vi "DestroyClone.vi"(8 "error in (no error)":errorcluster, 9 "Exit via Stop Module Req?":bool, 10 "Wait for Module to stop?":bool, 11 "ModuleAdmin":refnum<class "ModuleAdmin.lvclass">) -> (0 "error out":errorcluster, 1 "External Launch":bool, 3 "Mod Admin out":refnum<class "ModuleAdmin.lvclass">)   [LabVIEW 2014, in "SamplerModule.lvlib"]
uses:
  SamplerModule.lvlib
  <userlib>/NIST/ModuleAdminLib/ModuleAdmin/ModuleAdmin.lvclass
  <userlib>/NIST/ModuleAdminLib/ModuleAdmin/ModuleAdmin.lvclass/ModuleAdmin.ctl
  <userlib>/NIST/ModuleAdminLib/ModuleAdmin/Accessors/Read CloneRegRef.vi
  <userlib>/NIST/ModuleAdminLib/CloneRegistration/CloneRegistration.lvclass
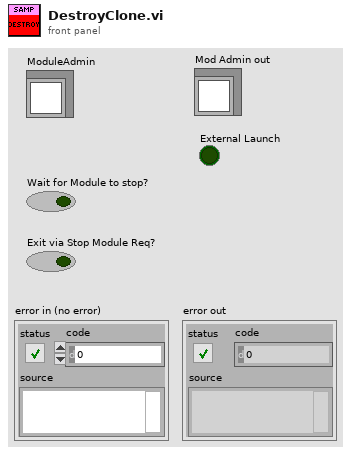
[diagram p1: front panel]
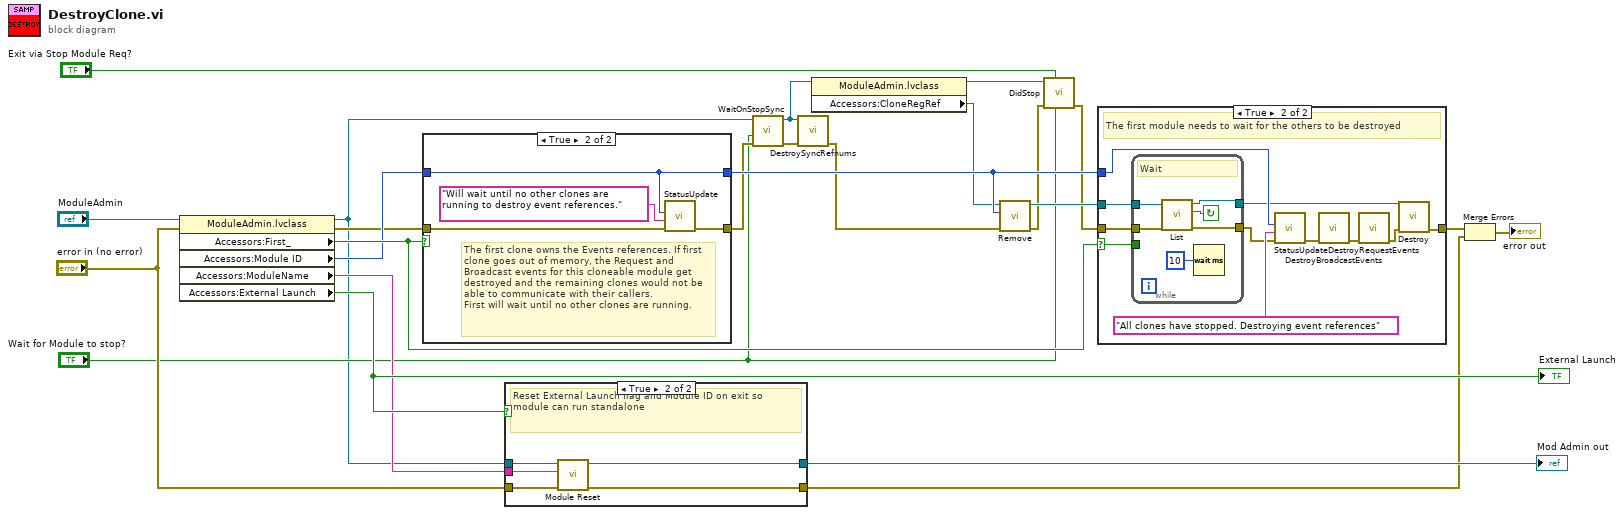
[diagram p0: block diagram]
diagram:
  n1 = property class="ModuleAdmin.lvclass"(reference="ModuleAdmin", error in="error in (no error)") -> (reference out=w2:refnum<class "ModuleAdmin.lvclass">, error out=w11:errorcluster, "Accessors:First_"=w24:bool, "Accessors:Module ID"=w15:i32, "Accessors:ModuleName"=w19:string, "Accessors:External Launch"=w21:bool)
  "External Launch" <- w21
  n2 = case shown="True" w24 {
    tunnel: w11 -> [w26 w30]
    tunnel: w15 -> [w25 w27]
    tunnel: [w26 w28] -> w10
    tunnel: [w25 w27] -> w23
    frame False {
    }
    frame True {
      # "The first clone owns the Events references. If first clone goes out of memory, the Request and Broadcast events for this cloneable module get destroyed and the remaining clones would not be able to communicate with their callers.\nFirst will wait until no other clones are running."
      n3 = call "StatusUpdate.vi"("error in (no error)"=w30, "Status"="Will wait until no other clones are running to destroy event references." ("format string"), "ModuleID"=w27) -> ("error out"=w28:errorcluster)  [unwired: 8 in]
    }
  }
  n4 = case shown="True" w21 {
    tunnel: "error in (no error)" -> [w31 w37]
    tunnel: w19 -> [_ w36]
    tunnel: w2 -> [w32 w35]
    tunnel: [w32 w34] -> w18
    tunnel: [w31 w33] -> w16
    frame False {
    }
    frame True {
      # "Reset External Launch flag and Module ID on exit so module can run standalone"
      n5 = call <userlib>:"Module Reset.vi"("error in (no error)"=w37, "ModuleName"=w36, "Mod Admin in"=w35) -> ("error out"=w33:errorcluster, "Mod Admin out"=w34:refnum<class "ModuleAdmin.lvclass">)  [unwired: 7 in]
    }
  }
  "Mod Admin out" <- w18
  n6 = call <userlib>:"WaitOnStopSync.vi"("error in (no error)"=w10, "WaitForModuleToStop?"="Wait for Module to stop?", "ModuleAdmin"=w2) -> ("error out"=w22:errorcluster, "ModuleAdmin"=w9:refnum<class "ModuleAdmin.lvclass">)  [unwired: 7 in]
  n7 = call <userlib>:"DestroySyncRefnums.vi"("error in (no error)"=w22, "ModuleAdmin"=w9) -> ("error out"=w7:errorcluster)  [unwired: 9 in]
  n8 = property class="ModuleAdmin.lvclass"(reference=w9) -> (reference out=w6:refnum<class "ModuleAdmin.lvclass">, "Accessors:CloneRegRef"=w8:refnum<data-value>)  [unwired: 1 in, 1 out]
  n9 = call <userlib>:"Remove.vi"("error in (no error)"=w7, "Module ID"=w23, "CloneRegRef"=w8) -> ("error out"=w12:errorcluster, "CloneRegRef"=w14:refnum<data-value>)  [unwired: 6 in, 1 out]
  n10 = call "DidStop.vi"("Wait for Module to stop?"="Wait for Module to stop?", "Exit via Stop Module Req?"="Exit via Stop Module Req?", "error in (no error)"=w12, "ModuleAdmin"=w6) -> ("error out"=w3:errorcluster)  [unwired: 7 in]
  n11 = case shown="True" w24 {
    selector: w24 -> [_ w48]
    tunnel: w3 -> [w38 w49]
    tunnel: w23 -> [_ w43]
    tunnel: [w38 w41] -> w13
    tunnel: w14 -> [_ w42]
    frame False {
    }
    frame True {
      # "The first module needs to wait for the others to be destroyed"
      n12 = while {
        tunnel: w49 -> [w55]
        tunnel: w48 -> [_]
        tunnel: [w54] -> w46
        tunnel: w42 -> [w51]
        tunnel: [w50] -> w40
        stop <- w53 continue-if-true
        # "Wait"
        n13 = call <userlib>:"List.vi"("error in (no error)"=w55, "CloneRegRef"=w51) -> ("error out"=w54:errorcluster, "Found?"=w53:bool, "CloneRegRef"=w50:refnum<data-value>)  [unwired: 4 in, 3 out]
        n14 = Wait (ms)(milliseconds to wait=u32 10) -> ()  [unwired: 1 out]
      }
      n15 = call "StatusUpdate.vi"("error in (no error)"=w46, "Status"="All clones have stopped. Destroying event references", "ModuleID"=w43) -> ("error out"=w45:errorcluster)  [unwired: 8 in]
      n16 = call "DestroyBroadcastEvents.vi"("error in (no error)"=w45) -> ("error out"=w44:errorcluster)  [unwired: 10 in]
      n17 = call "DestroyRequestEvents.vi"("error in (no error)"=w44) -> ("error out"=w39:errorcluster)  [unwired: 10 in]
      n18 = call <userlib>:"Destroy.vi"("error in (no error)"=w39, "CloneRegRef"=w40) -> ("error out"=w41:errorcluster)  [unwired: 9 in]
    }
  }
  n19 = Merge Errors(w13, w16) -> (→"error out":errorcluster)
